vi "Fit Model to Plot v3.vi"(0 "Fit Plot Information":T5={"XY Graph Ref"=refnum, "Mouse Coordinates"={"X"=0.0, "Y"=0.0}, "Fit Model"=enum."Select a Fit Model...", "Plot Index"=-1}, 5 "Fit Settings":T1={"Use Histogram # Points"=TRUE, "# Fit Plot Points"=0, "Fit Method"=0, "Weighted Histogram Fit"=FALSE, "Show All Fit Components"=FALSE, "Ramp Type"=0} {"Ramp Type" items=["Linear", "Logarithmic"]; "Fit Method" items=["Least Square", "Least Absolute Residual", "Bisquare"]}, 9 "Fixed Parameters":T4, 11 "error in (no error)":errorcluster, 12 "Bin Location":T8, 13 "Send Graph to Notebook?":bool) -> (1 "Fitted Plot":cluster{"X Array":dbl[], "Y Array":dbl[]}, 3 "Plot Name":string, 4 "Graph Caption":string, 6 "Fit Parameter Names":string[](array[string]), 10 "Fit Parameter Values":dbl[](array[numeric]), 14 "Fit Result String":string, 15 "error out":errorcluster)   [LabVIEW 2019]
uses:
  Histogram Bin Position.ctl
  Fit Plot Request Information.ctl
  <vilib>/Utility/miscctls.llb/LVPointDoubleTypeDef.ctl
  Fit Models.ctl
  D-Only Fixed Parameters.ctl
  Fit Settings.ctl
  <vilib>/Analysis/6fits.llb/Curve Fitting Criteria.ctl
  Ramp Type.ctl
  <vilib>/Analysis/NI_AALPro.lvlib
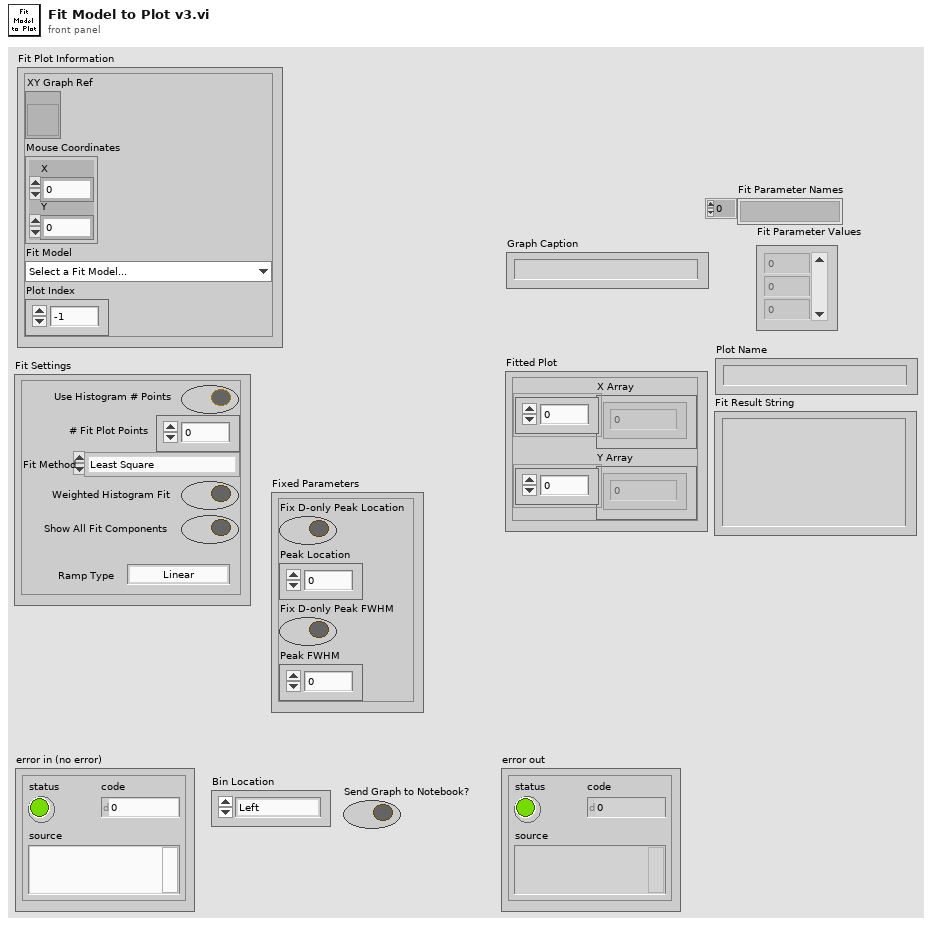
[diagram p1: front panel]
types:
  T1 = typedef "Fit Settings.ctl" = cluster{"Use Histogram # Points":bool, "# Fit Plot Points":u32, "Fit Method":T2, "Weighted Histogram Fit":bool, "Show All Fit Components":bool, "Ramp Type":T3}
  T2 = typedef "NI_AALPro.lvlib/Curve Fitting Criteria.ctl" = u16
  T3 = typedef "Ramp Type.ctl" = u16
  T4 = typedef "D-Only Fixed Parameters.ctl" = cluster{"Fix D-only Peak Location":bool, "Peak Location":dbl, "Fix D-only Peak FWHM":bool, "Peak FWHM":dbl}
  T5 = typedef "Fit Plot Request Information.ctl" = cluster{"XY Graph Ref":refnum<vi>, "Mouse Coordinates":T6, "Fit Model":T7, "Plot Index":i32}
  T6 = typedef "LVPointDoubleTypeDef.ctl" = cluster{"X":dbl, "Y":dbl}
  T7 = typedef "Fit Models.ctl" = enum16{"Select a Fit Model...", "           Single Peak", "Gaussian", "Asymmetric Gaussian", "Lorentzian", "Asymmetric Lorentzian", "Gaussian/Lorentzian", "Lorentzian/Gaussian", "           Double Peak", "Two Gaussians", "Two Asymmetric Gaussians", "Two H-Connected Gaussians", "Two T-Connected Gaussians", "Two H-Connected Asymmetric Gaussians", "Two T-Connected Asymmetric Gaussians", "           Triple Peak", "Three Gaussians", "Three Asymmetric Gaussians", "              Decays", "Single Exponential", "Two Exponentials", "               ACF", "2D Gaussian ACF", "2D Gaussian + Blinking ACF", "2D Gaussian + Flow ACF", "3D Gaussian ACF", "3D Gaussian + Blinking ACF", "             Multiplot", "2D Gaussian ACF & 2D Gaussian + Flow ACF"}
  T8 = typedef "Histogram Bin Position.ctl" = enum16{"Left", "Center", "Right"}
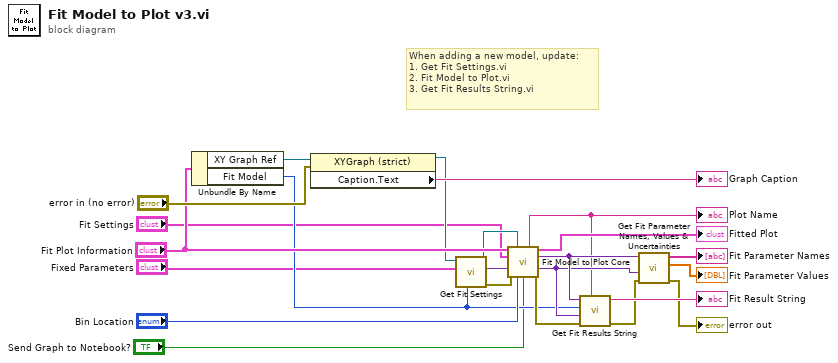
[diagram p0: block diagram]
diagram:
  # "When adding a new model, update:\n1. Get Fit Settings.vi\n2. Fit Model to Plot.vi\n3. Get Fit Results String.vi"
  n1 = Unbundle By Name("Fit Plot Information") -> ("XY Graph Ref"=w15:refnum<vi>, "Fit Model"=w6:T7)
  n2 = property class="XYGraph (strict)"(reference=w15, error in="error in (no error)") -> (reference out=w10:refnum<vi>, "Caption.Text"=→"Graph Caption":string)  [unwired: 1 out]
  n3 = call "Get Fit Settings.vi"("Fit Model"=w6, "Fixed Parameters"="Fixed Parameters", "XY Graph Ref"=w10) -> ("Error Out"=w2:errorcluster, "Additional Fit Settings"=w5:variant, "LM Function & Gradient"=w11:refnum<vi>)  [unwired: 6 in]
  n4 = call "Fit Model to Plot Core.vi"("Fit Plot Information"="Fit Plot Information", "LM Function & Gradient"=w11, "Fit Settings"="Fit Settings", "Additional Data"=w5, "error in (no error)"=w2, "Bin Location"="Bin Location", "Send Graph to Notebook?"="Send Graph to Notebook?") -> ("Plot Name"=w9:string, "Fitted Plot"=→"Fitted Plot":cluster{"X Array":dbl[], "Y Array":dbl[]}, "Fit Parameters Cluster"=w13:variant, "Fit Parameters Uncertainties Cluster"=w12:variant, "error out"=w8:errorcluster)  [unwired: 3 in, 1 out]
  "Plot Name" <- w9
  n5 = call "Get Fit Results String.vi"("Plot Name"=w9, "error in (no error)"=w8, "Fit Parameters Uncertainties Cluster"=w12, "Fit Model"=w6, "Fit Parameters Cluster"=w13) -> ("error out"=w21:errorcluster, "Fit Results String"=→"Fit Result String":string)  [unwired: 5 in]
  n6 = call "Get Fit Parameter Names, Values & Uncertainties.vi"("error in (no error)"=w21, "Fit Parameter Uncertainties"=w12, "Fit Parameters"=w13) -> ("Error Out"=→"error out":errorcluster, "Fit Parameter Values"=→"Fit Parameter Values":dbl[], "Fit Parameter Names"=→"Fit Parameter Names":string[])  [unwired: 5 in, 1 out]
